vi "Configure Marker Frequency.vi"(8 "error in (no error)":errorcluster, 9 "Marker Frequency":dbl, 10 "Marker Number":u8=1, 11 "VNA-PNA in":refnum<class "VNA-PNA.lvclass">) -> (0 "error out":errorcluster, 3 "VNA-PNA out":refnum<class "VNA-PNA.lvclass">)   [LabVIEW 2020, in "VNA-PNA.lvclass"]
doc: "Configure the marker frequency.\nThe marker is always set on the current active trace."
uses:
  VNA-PNA.lvclass
  C:/Sandbox/RF Bench/Source Code/WiSpry Test Framework/Instruments/Instrument.lvclass
  Instrument.lvclass/Instrument.ctl
  Instrument.lvclass
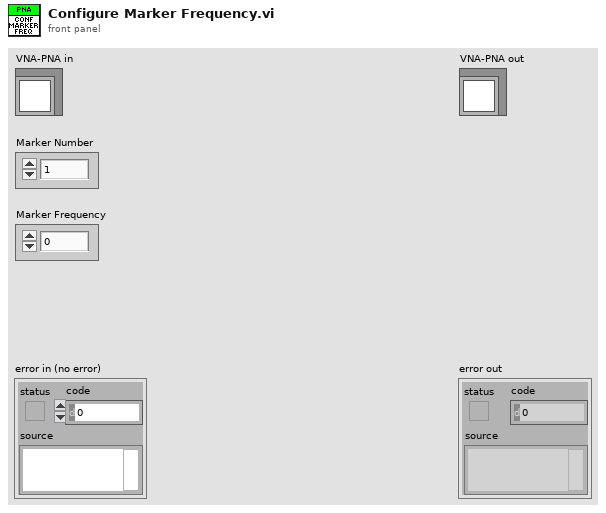
[diagram p1: front panel]
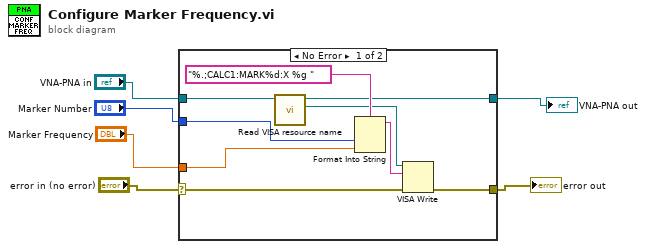
[diagram p0: block diagram]
diagram:
  n1 = case shown="No Error" "error in (no error)" {
    selector: "error in (no error)" -> [w14 w16]
    tunnel: "VNA-PNA in" -> [w15 w17]
    tunnel: "Marker Number" -> [w12 _]
    tunnel: "Marker Frequency" -> [w11 _]
    tunnel: [w8 w16] -> w1
    tunnel: [w7 w17] -> w2
    frame No Error {
      n2 = call "Read VISA resource name.vi"("Instrument in"=w15) -> ("VISA resource name"=w10:refnum<visa-resource-name>, "Instrument out"=w7:refnum<class "VNA-PNA.lvclass">)  [unwired: 9 in]
      n3 = Format Into String(format string="%.;CALC1:MARK%d:X %g ", w12, w11) -> (resulting string=w9:string)  [unwired: 2 in, 1 out]
      n4 = VISA Write(VISA resource name=w10, write buffer=w9, error in (no error)=w14) -> (error out=w8:errorcluster)  [unwired: 2 out]
    }
    frame Error {
    }
  }
  "error out" <- w1
  "VNA-PNA out" <- w2
